vi "Check Close.vi"(11 "Communication in":refnum<class "Communication.lvclass">) -> (4 "Stop?":bool)   [LabVIEW 2024, in "Communication.lvclass"]
doc: "MIT Licence\nCopyright (c) 2024 David Grollier"
uses:
  Communication.lvclass
  Communication.lvclass/Communication.ctl
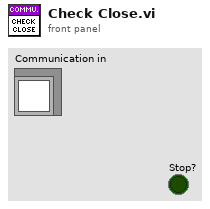
[diagram p1: front panel]
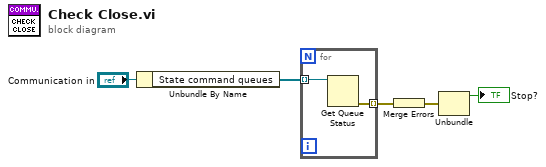
[diagram p0: block diagram]
diagram:
  n1 = Unbundle By Name("Communication in") -> ("State command queues"=w4:refnum<queue>[])
  n2 = for {
    tunnel: w4 -> [w7] mode=indexing
    tunnel: [w6] -> w3 mode=indexing
    n3 = Get Queue Status(queue=w7) -> (error out=w6:errorcluster)  [unwired: 2 in, 7 out]
  }
  n4 = Merge Errors(w3) -> (w2:errorcluster)
  n5 = Unbundle(w2) -> ("status"=→"Stop?":bool)  [unwired: 2 out]
